vi "Wavelet Transform Daubechies4 Inverse.vi"(0 "X":dbl[](array[numeric])) -> (1 "Wavelet Daubechies4 Inv {X}":dbl[](array[numeric]), 2 "error":i32)   [LabVIEW 2017, in "NI_Gmath.lvlib"]
doc: "Computes the inverse of the wavelet transform based on the Daubechies4 function of the input sequence <B>X</B>."
uses:
  NI_Gmath.lvlib
  Real Dot Product.vi
  NI_AALBase.lvlib
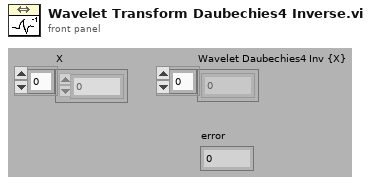
[diagram p1: front panel]
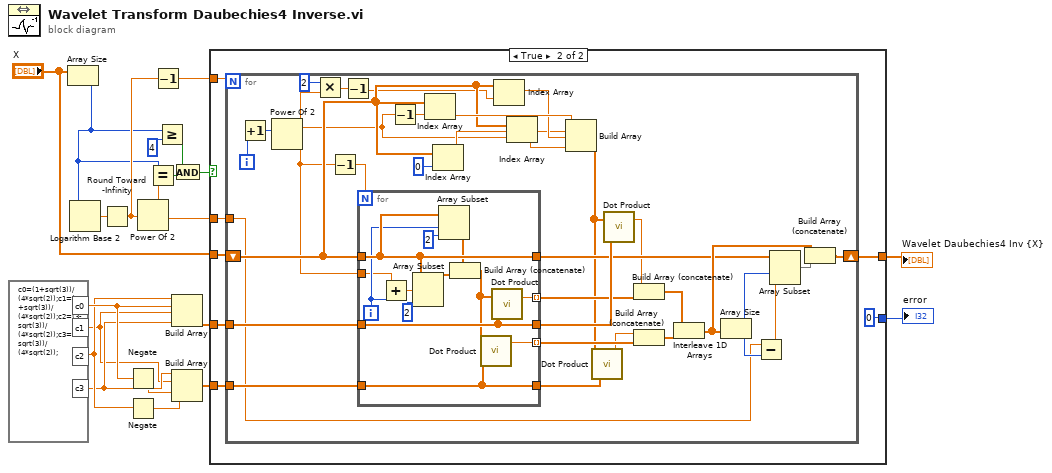
[diagram p0: block diagram]
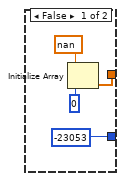
[diagram p2: hidden frame]
diagram:
  n1 = formula code="c0=(1+sqrt(3))/(4*sqrt(2));c1=(3+sqrt(3))/(4*sqrt(2));c2=(3-sqrt(3))/(4*sqrt(2));c3=(1-sqrt(3))/(4*sqrt(2));"() -> ("c0"=w11:dbl, "c1"=w8:dbl, "c2"=w10:dbl, "c3"=w9:dbl)
  n2 = Array Size(array="X") -> (size(s)=w3:i32)
  n3 = Logarithm Base 2(1:w3) -> (0:w20:dbl)
  n4 = Round Toward -Infinity(1:w20) -> (0:w5:dbl)
  n5 = Negate(x=w11) -> (-x=w7:dbl)
  n6 = Negate(x=w10) -> (-x=w6:dbl)
  n7 = Power Of 2(x=w5) -> (2^x=w19:dbl)
  n8 = Equal?(x=w3, y=w19) -> (x = y?=w15:bool)
  n9 = Decrement(x=w5) -> (x-1=w2:dbl)
  n10 = Greater Or Equal?(x=w3, y=4) -> (x >= y?=w16:bool)
  n11 = Build Array(w10, w11, w8, w9) -> (w13:dbl[])
  n12 = Build Array(w9, w8, w7, w6) -> (w12:dbl[])
  n13 = And(x=w16, y=w15) -> (x .and. y?=w14:bool)
  n14 = case shown="True" w14 {
    tunnel: [-23053 0] -> w18
    tunnel: w2 -> [_ w25]
    tunnel: "X" -> [_ w30]
    tunnel: w13 -> [_ w29]
    tunnel: w12 -> [_ w28]
    tunnel: w19 -> [_ w27]
    tunnel: [w21 w26] -> w1
    frame False {
      n15 = Initialize Array(nan, 0) -> (w21:dbl[])
    }
    frame True {
      n16 = for {
        N: w25 -> [_]
        shift-right: [w35] -> w26
        shift-left: w30 -> [w42]
        tunnel: w29 -> [w63]
        tunnel: w28 -> [w62]
        tunnel: w27 -> [w41]
        i -> [w33]
        n17 = Increment(x=w33) -> (x+1=w32:i32)
        n18 = Power Of 2(x=w32) -> (2^x=w34:dbl)
        n19 = Multiply(x=2, y=w34) -> (x*y=w38:dbl)
        n20 = Decrement(x=w34) -> (x-1=w43:dbl)
        n21 = Decrement(x=w38) -> (x-1=w36:dbl)
        n22 = for {
          N: w43 -> [_]
          tunnel: w42 -> [w72]
          tunnel: w63 -> [w75]
          tunnel: w62 -> [w74]
          tunnel: [w72] -> w56
          tunnel: [w75] -> w61
          tunnel: [w74] -> w60
          tunnel: [w68] -> w50 mode=indexing
          tunnel: [w67] -> w49 mode=indexing
          tunnel: w34 -> [w65]
          i -> [w66]
          n23 = Add(x=w65, y=w66) -> (x+y=w64:dbl)
          n24 = Array Subset(array=w72, index=w64, length=2) -> (w70:dbl[])
          n25 = Array Subset(array=w72, index=w66, length=2) -> (w71:dbl[])
          n26 = Build Array (concatenate)(w71, w70) -> (w69:dbl[])
          n27 = call-poly "Dot Product.vi"("Y Vector"=w74, "X Vector"=w69) -> ("X * Y"=w67:dbl)  [unwired: 1 out]
          n28 = call-poly "Dot Product.vi"("Y Vector"=w75, "X Vector"=w69) -> ("X * Y"=w68:dbl)  [unwired: 1 out]
        }
        n29 = Decrement(x=w34) -> (x-1=w39:dbl)
        n30 = Index Array(array=w42, index=w39) -> (element=w54:dbl)
        n31 = Index Array(array=w42, index=0) -> (element=w45:dbl)
        n32 = Index Array(array=w42, index=w36) -> (element=w53:dbl)
        n33 = Index Array(array=w42, index=w34) -> (element=w52:dbl)
        n34 = Build Array(w54, w45, w53, w52) -> (w44:dbl[])
        n35 = call-poly "Dot Product.vi"("Y Vector"=w60, "X Vector"=w44) -> ("X * Y"=w48:dbl)  [unwired: 1 out]
        n36 = call-poly "Dot Product.vi"("Y Vector"=w61, "X Vector"=w44) -> ("X * Y"=w51:dbl)  [unwired: 1 out]
        n37 = Build Array (concatenate)(w51, w50) -> (w47:dbl[])
        n38 = Build Array (concatenate)(w48, w49) -> (w46:dbl[])
        n39 = Interleave 1D Arrays(w47, w46) -> (w58:dbl[])
        n40 = Array Size(array=w58) -> (size(s)=w57:i32)
        n41 = Subtract(x=w41, y=w57) -> (x-y=w40:dbl)
        n42 = Array Subset(array=w56, index=w57, length=w40) -> (w59:dbl[])
        n43 = Build Array (concatenate)(w58, w59) -> (w35:dbl[])
      }
    }
  }
  "error" <- w18
  "Wavelet Daubechies4 Inv {X}" <- w1
